vi "GVECDs_ECD.vi"() -> ()   [LabVIEW 2017]
panel:
  out "ECD2Empfangen?":bool
  out "ECD1Empfangen?":bool
  out "ECD2MW":dbl[](array[numeric])
  out "ECD1MW":dbl[](array[numeric])
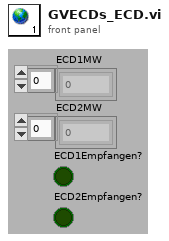
[diagram p1: front panel]
diagram:
